vi "zad4.vi"() -> ()   [LabVIEW 2025]
panel:
  out "Waveform Graph":dbl[][](graph)
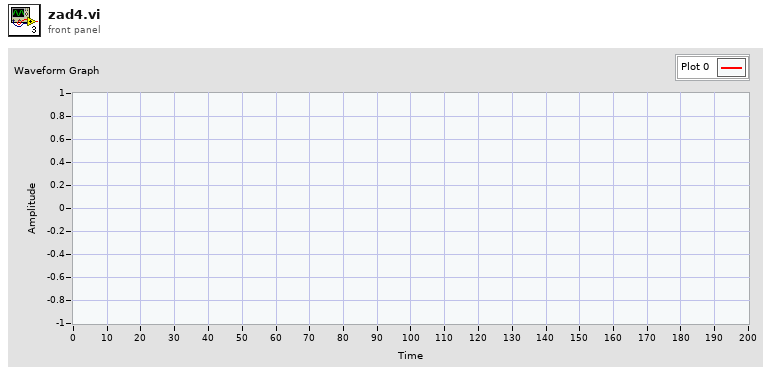
[diagram p1: front panel]
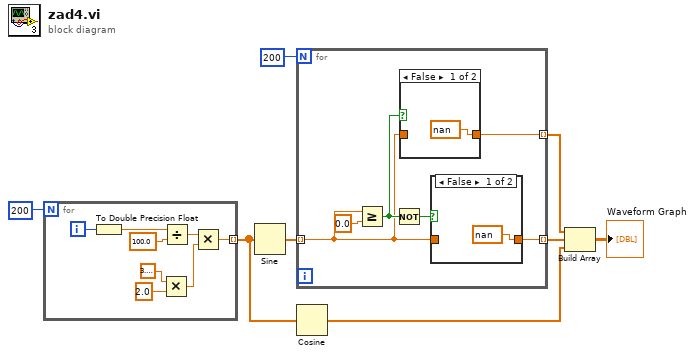
[diagram p0: block diagram]
diagram:
  n1 = for {
    N: 200 -> [_]
    tunnel: [w9] -> w2 mode=indexing
    i -> [w16]
    n2 = To Double Precision Float(number=w16) -> (double precision float=w15:dbl)
    n3 = Multiply(x=3.141592653589793, y=2.0) -> (x*y=w10:dbl)
    n4 = Divide(x=w15, y=100.0) -> (x/y=w13:dbl)
    n5 = Multiply(x=w13, y=w10) -> (x*y=w9:dbl)
  }
  n6 = Sine(x=w2) -> (sin(x)=w7:dbl[])
  n7 = for {
    N: 200 -> [_]
    tunnel: w7 -> [w18] mode=indexing
    tunnel: [w21] -> w5 mode=indexing
    tunnel: [w17] -> w4 mode=indexing
    n8 = Greater Or Equal?(x=w18, y=0.0) -> (x >= y?=w20:bool)
    n9 = Not(x=w20) -> (.not. x?=w19:bool)
    n10 = case shown="False" w20 {
      tunnel: w18 -> [_ w26]
      tunnel: [nan w26] -> w21
      frame False {
      }
      frame True {
      }
    }
    n11 = case shown="False" w19 {
      tunnel: w18 -> [_ w24]
      tunnel: [nan w24] -> w17
      frame False {
      }
      frame True {
      }
    }
  }
  n12 = Cosine(x=w2) -> (cos(x)=w1:dbl[])
  n13 = Build Array(w5, w4, w1) -> (→"Waveform Graph":dbl[][])
